vi "Debugger.vi"() -> ()   [LabVIEW 2016]
uses:
  grsim/grSim Robot Command.ctl
  <extravilib>/ChannelInstances/Lossy Stream-a[.](u8)/Read With Abort.vi
  <extravilib>/ChannelInstances/Lossy Stream-a[.](u8)/Write With Abort.vi
  <extravilib>/ChannelInstances/Lossy Stream-a[.](u8)/Endpoint.vi
  <vilib>/Instr/_visa.llb/VISA Configure Serial Port (Instr).vi
  <extravilib>/ChannelInstances/Lossy Stream-a[.](u8)/Instantiate.vi
  <extravilib>/ChannelInstances/Lossy Stream-a[.](u8)/)Channel.vi
  <resource>/ChannelSupport/_ChannelSupport/WaitIfNeeded.vi
  <extravilib>/ChannelInstances/Lossy Stream-a[.](u8).lvlib
panel:
  out "Robot cluster":T1
  out "read buffer":string
  in  "VISA resource name":refnum<visa-resource-name>
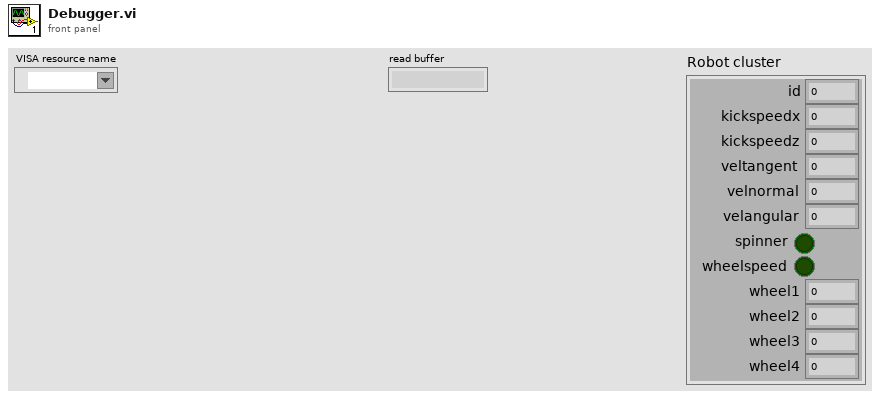
[diagram p1: front panel]
types:
  T1 = typedef "grSim Robot Command.ctl" = cluster{"id":u32, "kickspeedx":sgl, "kickspeedz":sgl, "veltangent":sgl, "velnormal":sgl, "velangular":sgl, "spinner":bool, "wheelspeed":bool, "wheel1":sgl, "wheel2":sgl, "wheel3":sgl, "wheel4":sgl}
  T2 = typedef "Lossy Stream-a[.](u8).lvlib/)Channel.ctl" = refnum<queue>
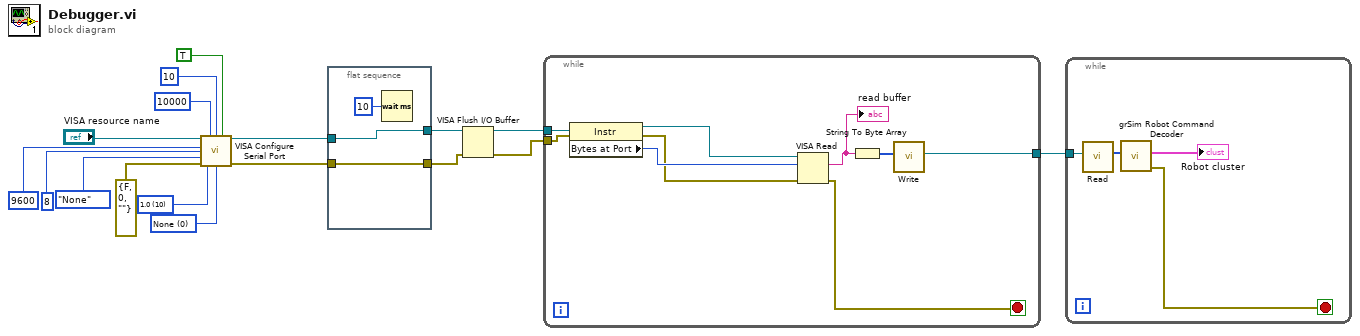
[diagram p0: block diagram]
diagram:
  w4 = u16 0 items=["None", "XON/XOFF", "RTS/CTS", "XON/XOFF & RTS/CTS", "DTR/DSR", "XON/XOFF & DTR/DSR"] ("flow control (0:none)")
  w5 = u16 10 items=["1.0"=10, "1.5"=15, "2.0"=20] ("stop bits (10: 1 bit)")
  n1 = call-poly "VISA Configure Serial Port"("VISA resource name"="VISA resource name", "timeout (10sec)"=u32 10000, "termination char\n(0xA = '\\n' = LF)"=u8 10 ("termination char\n(0xA = '\\n' = LF)"), "Enable Termination\nChar (T)"=TRUE ("Enable Termination\nChar (T)"), "baud rate (9600)"=u32 9600, "data bits (8)"=u16 8, "parity (0:none)"=enum16{"None", "Odd", "Even", "Mark", "Space"}."None", "error in (no error)"=errorcluster {"status"=FALSE, "code"=0, "source"=""}, "stop bits (10: 1 bit)"=w5, "flow control (0:none)"=w4) -> ("VISA resource name out"=w15:refnum<visa-resource-name>, "error out"=w13:errorcluster)  [unwired: 4 in]
  n2 = flat-sequence {
    tunnel: [w19] -> w16
    tunnel: w15 -> [w19]
    tunnel: [w18] -> w14
    tunnel: w13 -> [w18]
    frame #0 {
      n3 = Wait (ms)(milliseconds to wait=u32 10) -> ()  [unwired: 1 out]
    }
  }
  n4 = VISA Flush I/O Buffer(VISA resource name=w16, error in (no error)=w14) -> (VISA resource name out=w12:refnum<visa-resource-name>, error out=w11:errorcluster)  [unwired: 1 in]
  n5 = while {
    tunnel: w12 -> [w28]
    tunnel: [w24] -> w17
    tunnel: w11 -> [w22]
    stop <- w29 stop-if-true
    n6 = property class="Instr"(reference=w28, error in=w22) -> (reference out=w27:refnum<visa-resource-name>, error out=w21:errorcluster, "Bytes at Port"=w26:u32)
    n7 = VISA Read(VISA resource name=w27, byte count=w26, error in (no error)=w21) -> (read buffer=w23:string, error out=w29:errorcluster)  [unwired: 2 out]
    "read buffer" <- w23
    n8 = String To Byte Array(string=w23) -> (unsigned byte array=w25:u8[])
    n9 = call <extravilib>:"Write.vi"("element"=w25) -> ("channel"=w24:T2)  [unwired: 8 in, 2 out]
  }
  n10 = while {
    tunnel: w17 -> [w33]
    stop <- w32 stop-if-true
    n11 = call <extravilib>:"Read.vi"("channel"=w33) -> ("element"=w31:u8[])  [unwired: 5 in, 5 out]
    n12 = call "grSim Robot Command Decoder.vi"("Array"=w31) -> ("error out"=w32:errorcluster, "Robot cluster"=→"Robot cluster":T1)  [unwired: 8 in, 1 out]
  }
